vi "#178_MAV_MSG_AHRS2_DECODE.vi"(11 "mavlink_payload":u8[](array[numeric])) -> (3 "AHRS2":T1)   [LabVIEW 2023]
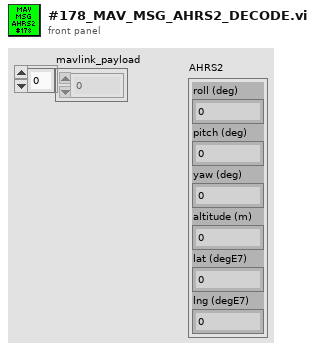
[diagram p1: front panel]
types:
  T1 = cluster{"roll (deg)":sgl, "pitch (deg)":sgl, "yaw (deg)":sgl, "altitude (m)":sgl, "lat (degE7)":i32, "lng (degE7)":i32}
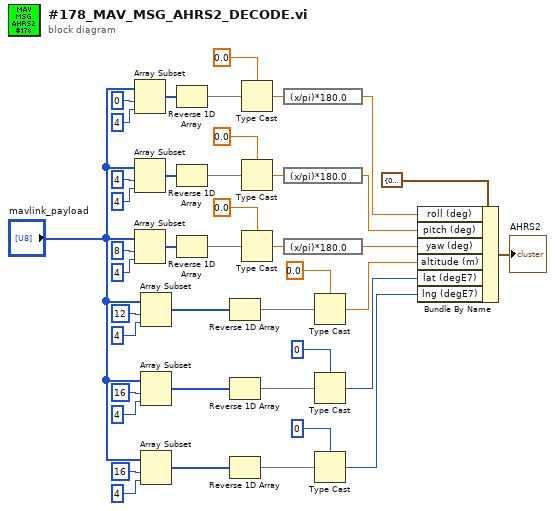
[diagram p0: block diagram]
diagram:
  n1 = Array Subset(array="mavlink_payload", index=0 ("Index"), length=4) -> (w41:u8[])
  n2 = Array Subset(array="mavlink_payload", index=4 ("Index"), length=4) -> (w32:u8[])
  n3 = Array Subset(array="mavlink_payload", index=8 ("Index"), length=4) -> (w26:u8[])
  n4 = Array Subset(array="mavlink_payload", index=12 ("Index"), length=4) -> (w20:u8[])
  n5 = Array Subset(array="mavlink_payload", index=16 ("Index"), length=4) -> (w15:u8[])
  n6 = Array Subset(array="mavlink_payload", index=16 ("Index"), length=4) -> (w6:u8[])
  n7 = Reverse 1D Array(array=w41) -> (reversed array=w40:u8[])
  n8 = Reverse 1D Array(array=w32) -> (reversed array=w31:u8[])
  n9 = Reverse 1D Array(array=w26) -> (reversed array=w25:u8[])
  n10 = Reverse 1D Array(array=w20) -> (reversed array=w19:u8[])
  n11 = Reverse 1D Array(array=w15) -> (reversed array=w14:u8[])
  n12 = Reverse 1D Array(array=w6) -> (reversed array=w5:u8[])
  n13 = Type Cast(type=sgl 0.0 ("Index"), x=w40) -> (*(type *) &x=w37:sgl)
  n14 = Type Cast(type=sgl 0.0 ("Index"), x=w31) -> (*(type *) &x=w28:sgl)
  n15 = Type Cast(type=sgl 0.0 ("Index"), x=w25) -> (*(type *) &x=w22:sgl)
  n16 = expression code="(x/pi)*180.0" ("radians to degrees")(w37) -> (w34:sgl)
  n17 = expression code="(x/pi)*180.0" ("radians to degrees")(w28) -> (w11:sgl)
  n18 = expression code="(x/pi)*180.0" ("radians to degrees")(w22) -> (w10:sgl)
  n19 = Type Cast(type=sgl 0.0 ("Index"), x=w19) -> (*(type *) &x=w9:sgl)
  n20 = Type Cast(type=0 ("Index"), x=w14) -> (*(type *) &x=w8:i32)
  n21 = Type Cast(type=0 ("Index"), x=w5) -> (*(type *) &x=w1:i32)
  n22 = Bundle By Name(cluster=T1 {"roll (deg)"=0.0, "pitch (deg)"=0.0, "yaw (deg)"=0.0, "altitude (m)"=0.0, "lat (degE7)"=0, "lng (degE7)"=0} ("AHRS2"), "roll (deg)"=w34, "pitch (deg)"=w11, "yaw (deg)"=w10, "altitude (m)"=w9, "lat (degE7)"=w8, "lng (degE7)"=w1) -> (→"AHRS2":T1)
